vi "FindOPCDLLPath.vi"() -> (3 "DLL Path":path)   [LabVIEW 2019]
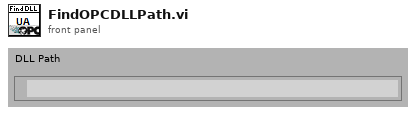
[diagram p1: front panel]
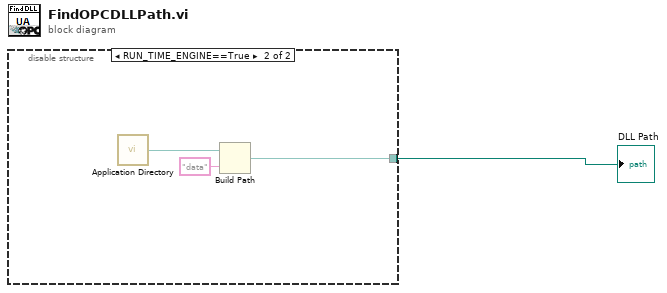
[diagram p0: block diagram]
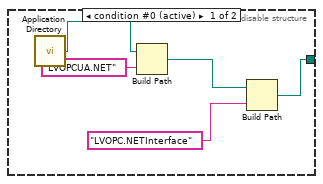
[diagram p2: hidden frame]
diagram:
  n1 = disable-structure shown="RUN_TIME_ENGINE==True" {
    disable-tunnel: [w2 w7] -> w1
    frame condition #0 (active) {
      n2 = call <vilib>:"Application Directory.vi"() -> ("Application Directory"=w5:path)
      n3 = Build Path(base path=w5, name or relative path="LVOPCUA.NET") -> (appended path=w4:path)
      n4 = Build Path(base path=w4, name or relative path="LVOPC.NETInterface") -> (appended path=w2:path)
    }
    frame condition #1 {
      n5 = call <vilib>:"Application Directory.vi"() -> ("Application Directory"=w8:path)
      n6 = Build Path(base path=w8, name or relative path="data") -> (appended path=w7:path)
    }
  }
  "DLL Path" <- w1
